vi "Write Sinewave Signal Samples to File 1.vi"() -> ()   [LabVIEW 2014]
uses:
  <vilib>/LabVIEW Universal Transcriptor/LabVIEW to Arduino Transcriptor/Transcriptors/System API/Serial println string.vi
  <vilib>/LabVIEW Universal Transcriptor/LabVIEW Universal Transcriptor SD Card Library/File Class/write float.vi
  <vilib>/LabVIEW Universal Transcriptor/LabVIEW to Arduino Transcriptor/Transcriptors/System API/Serial print string.vi
  <vilib>/measure/maspectr.llb/FFT Spectrum (Mag-Phase) for 1 Chan.vi
  <vilib>/LabVIEW Universal Transcriptor/LabVIEW Universal Transcriptor SD Card Library/File.lvclass
  <vilib>/LabVIEW Universal Transcriptor/LabVIEW Universal Transcriptor SD Card Library/LabVIEW Universal Transcriptor SD Card Library.lvlib
  <vilib>/LabVIEW Universal Transcriptor/LabVIEW to Arduino Transcriptor/Transcriptors/System API/System Serial Library Variables/System Serial Library Variables.lvlib
  <vilib>/LabVIEW Universal Transcriptor/LabVIEW for Arduino Math Library/Arduino Math.lvlib
  <vilib>/measure/NI_MAPro.lvlib
panel:
  out "DEBUG signal spectrum":cluster{"f0":dbl, "df":dbl, "magnitude":dbl[]}(graph)
  out "DEBUG signal output":sgl[](graph)
  out "String Buffer":string
  out "error out":errorcluster
  in  "Error In":errorcluster
  # "THIS WILL NOT APPEAR IN RESULT CODE\nit's inside enabled Diagram Disable Structure which is not generated into result code :)"
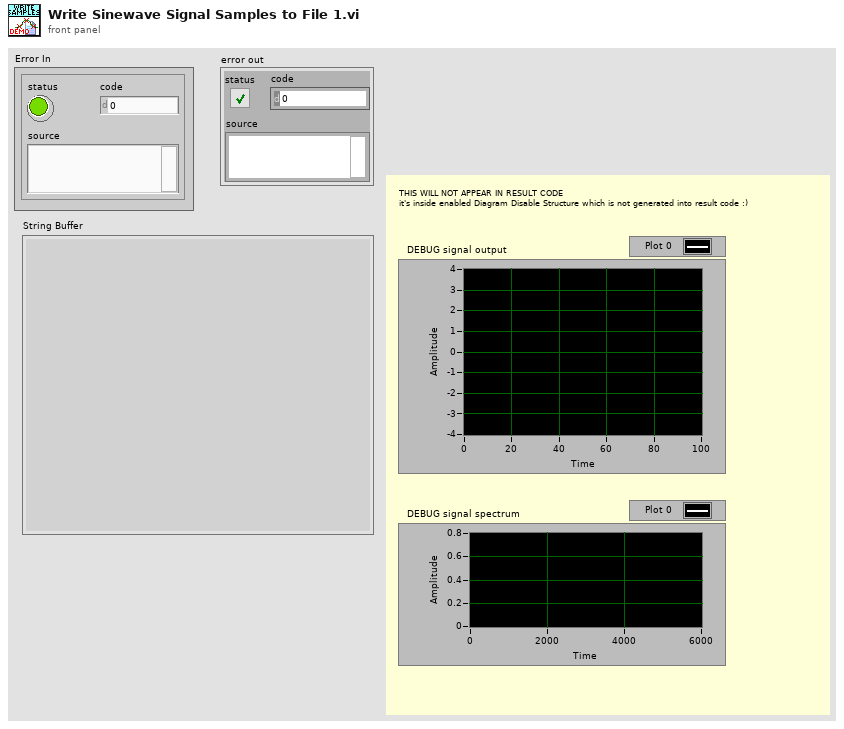
[diagram p1: front panel]
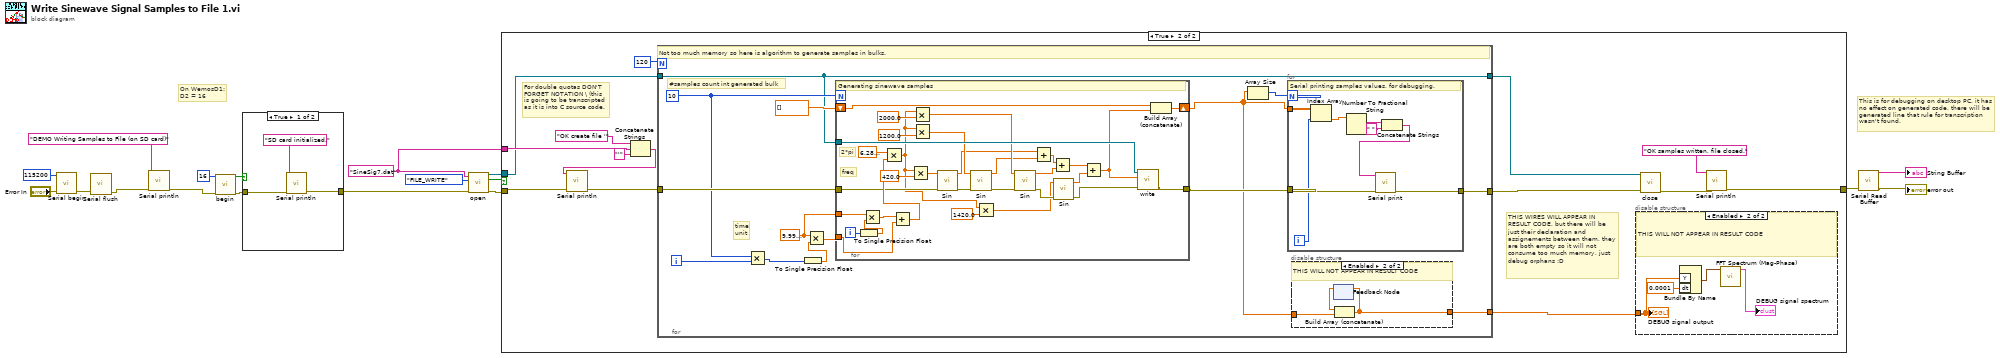
[diagram p0: block diagram]
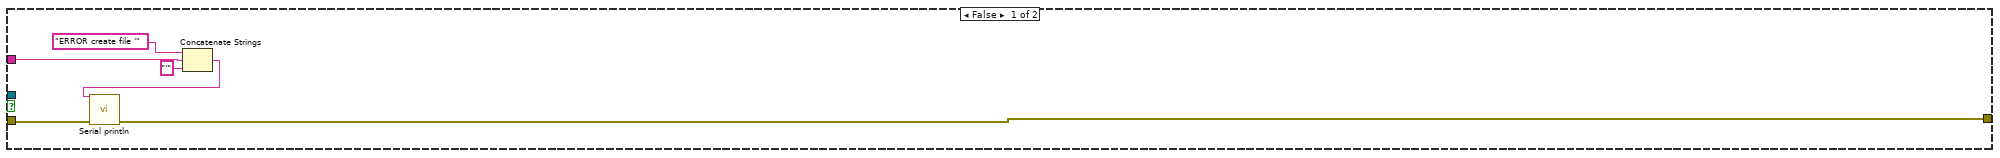
[diagram p2: hidden frame]
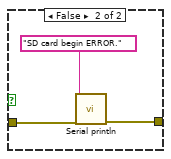
[diagram p5: hidden frame]
diagram:
  w1 = "SineSig7.dat" ("filepath")
  # "On WemosD1:\nD2 = 16"
  # "This is for debugging on desktop PC, it has\nno effect on generated code, there will be\ngenerated line that rule for transcription\nwasn't found."
  n1 = call <vilib>:"Serial begin.vi"("Error In"="Error In", "speed (Bd)"=115200) -> ("Error Out"=w18:errorcluster)  [unwired: 9 in]
  n2 = call <vilib>:"Serial flush.vi"("Error In"=w18) -> ("Error Out"=w16:errorcluster)  [unwired: 10 in]
  n3 = call-poly <vilib>:"Serial println.vi"("Error In"=w16, "string in"="DEMO Writing Samples to File (on SD card)") -> ("Error Out"=w14:errorcluster)  [unwired: 9 in]
  n4 = call <vilib>:"begin.vi"("Error In"=w14, "CS pin (optional)"=u8 16) -> ("Error Out"=w11:errorcluster, "success?"=w12:bool)  [unwired: 8 in]
  n5 = case shown="True" w12 {
    tunnel: w11 -> [w21 w24]
    tunnel: [w19 w22] -> w2
    frame True {
      n6 = call-poly <vilib>:"Serial println.vi"("Error In"=w21, "string in"="SD card initialized.") -> ("Error Out"=w19:errorcluster)  [unwired: 9 in]
    }
    frame False {
      n7 = call-poly <vilib>:"Serial println.vi"("Error In"=w24, "string in"="SD card begin ERROR.") -> ("Error Out"=w22:errorcluster)  [unwired: 9 in]
    }
  }
  n8 = call <vilib>:"open.vi"("Error In"=w2, "mode"=enum16{"FILE_READ", "FILE_WRITE"}."FILE_WRITE", "filepath"=w1) -> ("Error Out"=w9:errorcluster, "opened?"=w8:bool, "File out"=w7:refnum<class "File.lvclass">)  [unwired: 6 in]
  n9 = case shown="True" w8 {
    tunnel: w9 -> [w26 w41]
    tunnel: w1 -> [w30 w40]
    tunnel: [w25 w33] -> w6
    tunnel: w7 -> [_ w38]
    frame False {
      n10 = Concatenate Strings("ERROR create file '" ("string in"), w30, "'" ("string")) -> (w27:string)
      n11 = call-poly <vilib>:"Serial println.vi"("Error In"=w26, "string in"=w27) -> ("Error Out"=w25:errorcluster)  [unwired: 9 in]
    }
    frame True {
      # "THIS WIRES WILL APPEAR IN RESULT CODE, but there will be just their declaration and assignements between them, they are both empty so it will not consume too much memory, just debug orphans :D"
      # "For double quotas DON'T\nFORGET NOTATION \\ (this\nis going to be transcripted\nas it is into C source code."
      n12 = Concatenate Strings("OK create file '" ("string in"), w40, "'" ("string")) -> (w42:string)
      n13 = call-poly <vilib>:"Serial println.vi"("Error In"=w41, "string in"=w42) -> ("Error Out"=w39:errorcluster)  [unwired: 9 in]
      n14 = for {
        N: 120 -> [_]
        tunnel: w39 -> [w59]
        tunnel: w38 -> [w54]
        tunnel: [w54] -> w37
        tunnel: [w58] -> w32
        tunnel: [w49] -> w31
        i -> [w56]
        w51 = sgl 0.0001 ("x")
        w57 = 10
        # "#samples count int generated bulk"
        # "time\nunit"
        # "Not too much memory so here is algorithm to generate samples in bulks."
        n15 = Multiply(x=w57, y=w56) -> (x*y=w55:i32)
        n16 = To Single Precision Float(number=w55) -> (single precision float=w61:sgl)
        n17 = Multiply(x=w51, y=w61) -> (x*y=w60:sgl)
        n18 = for {
          N: w57 -> [_]
          tunnel: w59 -> [w95]
          shift-right: [w100] -> w50
          shift-left: sgl[] [] ("initialized array") -> [w101]
          tunnel: [w93] -> w53
          tunnel: w51 -> [w97]
          tunnel: w60 -> [w96]
          tunnel: w54 -> [w94]
          i -> [w105]
          # "freq"
          # "2*pi"
          # "Generating sinewave samples"
          n19 = To Single Precision Float(number=w105) -> (single precision float=w102:sgl)
          n20 = Multiply(x=w97, y=w102) -> (x*y=w99:sgl)
          n21 = Add(x=w99, y=w96) -> (x+y=w98:sgl)
          n22 = Multiply(x=sgl 6.28, y=w98) -> (x*y=w74:sgl)
          n23 = Multiply(x=w74, y=sgl 420.0) -> (x*y=w85:sgl)
          n24 = Multiply(x=w74, y=sgl 2000.0) -> (x*y=w87:sgl)
          n25 = Multiply(x=w74, y=sgl 1200.0) -> (x*y=w86:sgl)
          n26 = call <vilib>:"Sin.vi"("Error In"=w95, "x"=w85) -> ("Error Out"=w89:errorcluster, "sin(x)"=w84:sgl)  [unwired: 8 in]
          n27 = call <vilib>:"Sin.vi"("Error In"=w89, "x"=w86) -> ("Error Out"=w90:errorcluster, "sin(x)"=w83:sgl)  [unwired: 8 in]
          n28 = Multiply(x=w74, y=sgl 1420.0) -> (x*y=w75:sgl)
          n29 = call <vilib>:"Sin.vi"("Error In"=w90, "x"=w87) -> ("Error Out"=w79:errorcluster, "sin(x)"=w82:sgl)  [unwired: 8 in]
          n30 = Add(x=w84, y=w83) -> (x+y=w88:sgl)
          n31 = Add(x=w88, y=w82) -> (x+y=w80:sgl)
          n32 = call <vilib>:"Sin.vi"("Error In"=w79, "x"=w75) -> ("Error Out"=w78:errorcluster, "sin(x)"=w77:sgl)  [unwired: 8 in]
          n33 = Add(x=w80, y=w77) -> (x+y=w81:sgl)
          n34 = call-poly <vilib>:"write.vi"("error in (no error)"=w78, "number"=w81, "File in"=w94) -> ("error out"=w93:errorcluster)  [unwired: 8 in]
          n35 = Build Array (concatenate)(w101, w81) -> (w100:sgl[])
        }
        n36 = Array Size(array=w50) -> (size(s)=w52:i32)
        n37 = for {
          N: w52 -> [_]
          tunnel: w53 -> [w67]
          tunnel: w50 -> [w73]
          tunnel: [w66] -> w58
          i -> [w72]
          # "Serial printing samples values, for debugging."
          n38 = Index Array(array=w73, index=w72) -> (element=w71:sgl)
          n39 = Number To Fractional String(number=w71) -> (F-format string=w69:string)  [unwired: 3 in]
          n40 = Concatenate Strings(w69, " " ("element")) -> (w68:string)
          n41 = call-poly <vilib>:"Serial print.vi"("Error In"=w67, "string in"=w68) -> ("Error Out"=w66:errorcluster)  [unwired: 9 in]
        }
        n42 = disable-structure shown="Enabled" {
          disable-tunnel: w50 -> [_ w64]
          disable-tunnel: [_ w63] -> w49
          frame Disabled {
          }
          frame Enabled {
            # "THIS WILL NOT APPEAR IN RESULT CODE"
            n43 = feedback #1() -> (w65:sgl[])  [unwired: 1 in]
            n44 = Build Array (concatenate)(w65, w64) -> (w63:sgl[])
            n45 = feedback-in #1(w63) -> ()
          }
        }
      }
      n46 = disable-structure shown="Enabled" {
        disable-tunnel: w31 -> [_ w47]
        frame Disabled {
        }
        frame Enabled {
          # "THIS WILL NOT APPEAR IN RESULT CODE"
          n47 = Bundle By Name("Y"=w47, "dt"=0.0001) -> (w48:waveform(sgl))  [unwired: 1 in]
          n48 = call-poly <vilib>:"FFT Spectrum (Mag-Phase).vi"("time signal"=w48) -> ("magnitude"=→"DEBUG signal spectrum":cluster{"f0":dbl, "df":dbl, "magnitude":dbl[]})  [unwired: 6 in, 4 out]
          "DEBUG signal output" <- w47
        }
      }
      n49 = call-dynamic "close.vi"("error in (no error)"=w32, "File in"=w37) -> ("error out"=w34:errorcluster)  [unwired: 9 in]
      n50 = call-poly <vilib>:"Serial println.vi"("Error In"=w34, "string in"="OK samples written, file closed.") -> ("Error Out"=w33:errorcluster)  [unwired: 9 in]
    }
  }
  n51 = call <vilib>:"Serial Read Buffer.vi"("Error In"=w6) -> ("Error Out"=→"error out":errorcluster, "String Buffer"=→"String Buffer":string)  [unwired: 9 in]
